vi "ReadImageParameters_JSON.vi"(8 "error in":errorcluster, 11 "Default JSON\nVariant in":variant) -> (0 "error out":errorcluster, 1 "VCluster\n out":variant, 2 "Error Message":string, 3 "Camera Names":string[](array[string]))   [LabVIEW 2015, in "ZenGage v3.0 UI.lvclass"]
uses:
  ZenGage v3.0 UI.lvclass
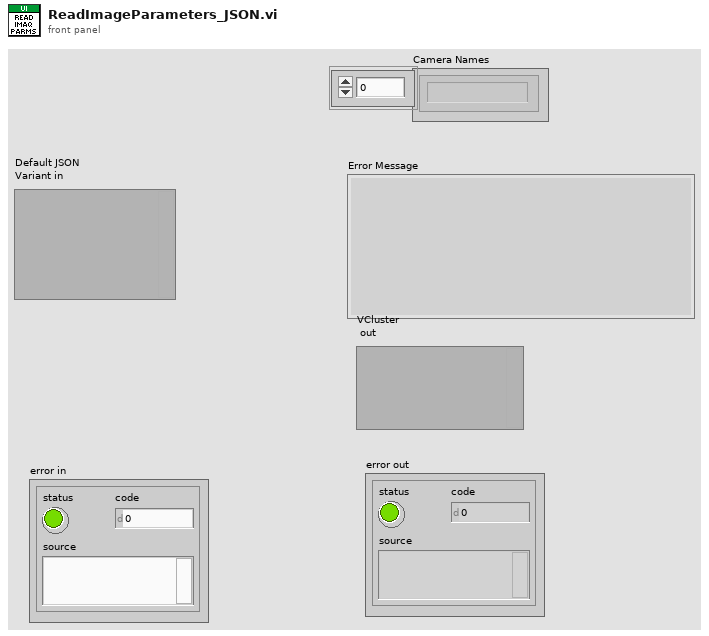
[diagram p1: front panel]
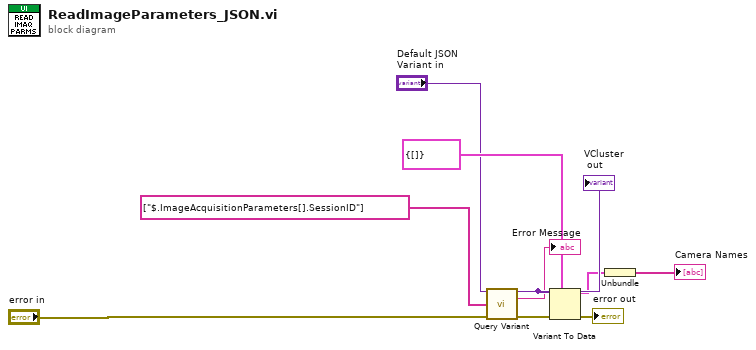
[diagram p0: block diagram]
diagram:
  n1 = call <vilib>:"Query Variant.vi"("VCluster in"="Default JSON\nVariant in", "pathList"=string[] ["$.ImageAcquisitionParameters[].SessionID"], "error IO"="error in") -> ("VCluster\n out"=w9:variant, "Error Message"=→"Error Message":string, "error out"=w5:errorcluster)  [unwired: 9 in, 1 out]
  "VCluster\n out" <- w9
  n2 = Variant To Data(error in=w5, type=cluster{string[]} {[]}, Variant=w9) -> (data=w3:cluster{string[]}, error out=→"error out":errorcluster)
  n3 = Unbundle(w3) -> (→"Camera Names":string[])
